vi "LET Output.vi"() -> ()   [LabVIEW 2010]
doc: "Cont(inuous) Acq(uire) & Chart (hw timed) demonstrates the hardware timed, non-buffered technique of data acquisition. The scan clock on the board controls acquisition timing. Acquired scans are read directly from the device's FIFO using AI Single Scan. \n\nThe acquisition is configured with no buffer, and the on-board scan clock started at the selected scan rate. In the first loop iteration, the newest (most recent) scan is read from the FIFO. In each subsequent loop iteration AI Single Scan is called to read the oldest scan from the FIFO. Then if a scan is missed because the acquisition does not keep up, an error message will be displayed, and the acquisition stopped. Each scan is plotted on the chart after it is read. \n\nA common reason to use non-buffered acquisition is that some kind of processing needs to be done for each data point. You will probably want to add more functions to the diagram to customize this VI for your application. The acquisition rate you can achieve depends on how much processing and display the VI must do. This VI calls a subVI named My Single-Scan Processing. Add whatever processing you need to this subVI, or replace it with one of your own. The data processing subVI also demonstrates how to use error clusters in your own subVIs, so they can be included in the error data flow chain.\n\nBefore running this VI, set the values of the controls on the front panel. Select Show Help Window from the Help menu to see a description of each control. If the values you select for all the controls are values you will usually use, select Make Current Values Default from the Operate menu and save the VI. Or, you may save individual control's default values by popping up on the control, selecting Data Operations, then selecting Make Current Value Default, and saving the VI."
uses:
  <instrlib>/agilent_b2900_series/Agilent B2900 Series/Public/Configure/Measurement/Configure Measurement (Current).vi
  <instrlib>/agilent_b2900_series/Agilent B2900 Series/Public/Configure/Measurement/Configure Measurement (Voltage).vi
  <vilib>/Analysis/Matrix/Numeric/Conversions/Matrix To Array - RM.vi
  <vilib>/Utility/file.llb/Write To Spreadsheet File (DBL).vi
  <vilib>/Utility/file.llb/Write To Spreadsheet File (string).vi
  <instrlib>/agilent_b2900_series/Agilent B2900 Series/Agilent B2900 Series.lvlib
  <vilib>/Analysis/Matrix/NI_Matrix.lvlib
panel:
  in  "File Name":string
  in  "WithTimeStamp":bool
  in  "File path":path
  in  "AutoSave":bool
  out "header":string[](array[string])
  out "Real 2D Array":dbl[][](array[numeric])
  out "data matrix":dbl[][](array[numeric])
  out "Igs array 2":dbl[][](array[numeric])
  out "Vgs array 2":dbl[][](array[numeric])
  out "Vds array 2":dbl[][](array[numeric])
  out "Corrected PD current array 2":dbl[][](array[numeric])
  out "Ids array 2":dbl[][](array[numeric])
  out "corrected PD current array":dbl[](array[numeric])
  out "Vds array":dbl[](array[numeric])
  out "Ids array":dbl[](array[numeric])
  out "Vgs array":dbl[](array[numeric])
  out "Igs array":dbl[](array[numeric])
  in  "Tab Control":T1(tab)
  in  "keithley address":string="GPIB0::20::INSTR"
  in  "agilent address":refnum<visa-resource-name>="GPIB0::23::INSTR"
  in  "Initial Vds (V)\n(100 scans/sec)":sgl caption="Initial Vds (V)" format="%.2f"
  in  "Vds step (V)":sgl=1.0 format="%.2f"
  in  "Vds delay time":sgl=10.0 caption="Vds delay time (ms)" format="%.2f"
  in  "Vds delay after first value (ms)":sgl=10.0 format="%.2f"
  in  "Final Vds(V)":sgl=60.0 format="%.2f"
  in  "light emission ON/OFF":bool=TRUE
  in  "Vgs step (V)":sgl=20.0 format="%.2f"
  in  "Final Vgs (V)":sgl=60.0 format="%.2f"
  in  "Initial Vgs (V)":sgl format="%.2f"
  in  "Vgs hold time (ms)":i32=10
  in  "Compliance Voltage (channel 2)":dbl=60.0
  in  "Compliance Current (channel 1)":dbl=0.001
  in  "Compliance Voltage (channel 1)":dbl=60.0
  in  "Compliance Current (channel 2)":dbl=0.0001
  in  "keithley compliance limit":dbl(ring)=0.025 items=["25uA"=2.5e-05, "250uA"=0.00025, "2.5mA"=0.0025, "25mA"=0.025]
  in  "Loop":bool=TRUE
  in  "keithley current resolution":dbl=0.01 format="%^.2e"
  in  "Current Auto Range Mode (0: Normal)":i32(ring) items=["Normal", "Resolution", "Speed"]
  in  "Voltage Auto Range Mode (0: Normal)":i32(ring) items=["Normal", "Resolution", "Speed"]
  out "Current Scan":cluster{dbl[], dbl[]}(graph)
  out "Applied Vds":sgl caption="current VDS (V)" format="%.2f"
  out "Applied Vgs":sgl caption="current VDS (V)" format="%.2f"
  out "Measured Ids":dbl format="%.2e"
  out "Measured Vds":dbl
  out "corrected PD current":dbl format="%^.2e"
  out "dark PD current (A)":dbl format="%^.2e"
  out "PD current":dbl format="%^.2e"
  out "Measured Igs":dbl
  out "Measured Vgs":dbl
  out "channel 2 status":bool
  out "channel 1 status":bool
  out "Current Scan 2":cluster{dbl[], dbl[]}(graph) caption="Current Scan"
  out "half  points":sgl
  out "Vds points":sgl
  out "Vgs points":sgl
  out "?":cluster{dbl[], dbl[]}[](graph)
  out "?":cluster{dbl[], dbl[]}[](graph)
  in  "error in keithley":errorcluster
  out "keithley address out":refnum<k15>
  out "error out keithley":errorcluster
  out "error out agilent":errorcluster
  out "Agilent address out":refnum<visa-resource-name>
  # "FET output v3"
  # "Drain-Source Setting"
  # "Gate Setting"
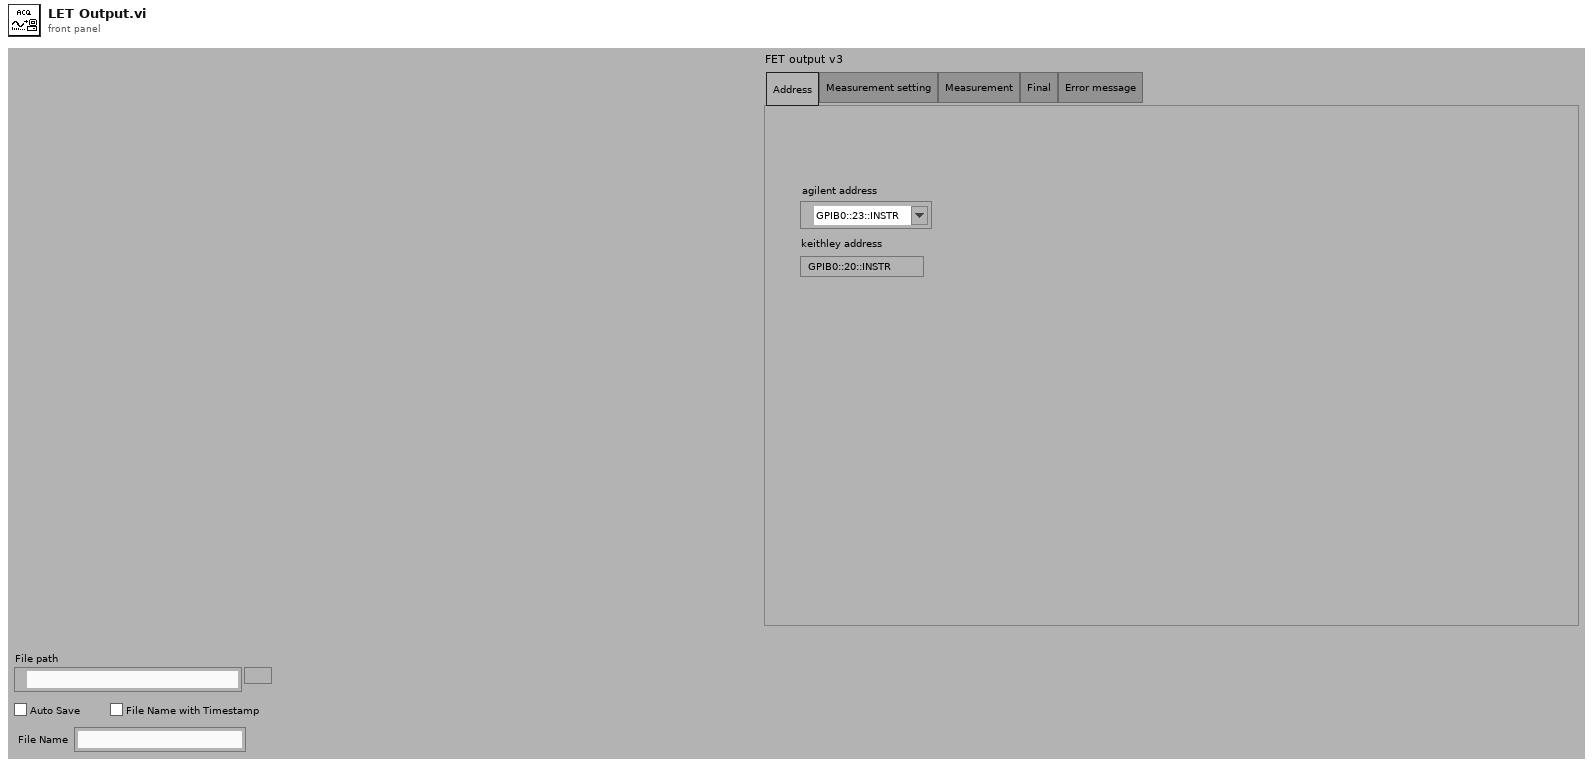
[diagram p1: front panel]
types:
  T1 = enum32{"Address", "Measurement setting", "Measurement", "Final", "Error message"}
  T2 = typedef "NI_Matrix.lvlib/RealMatrix.ctl" = dbl[][]
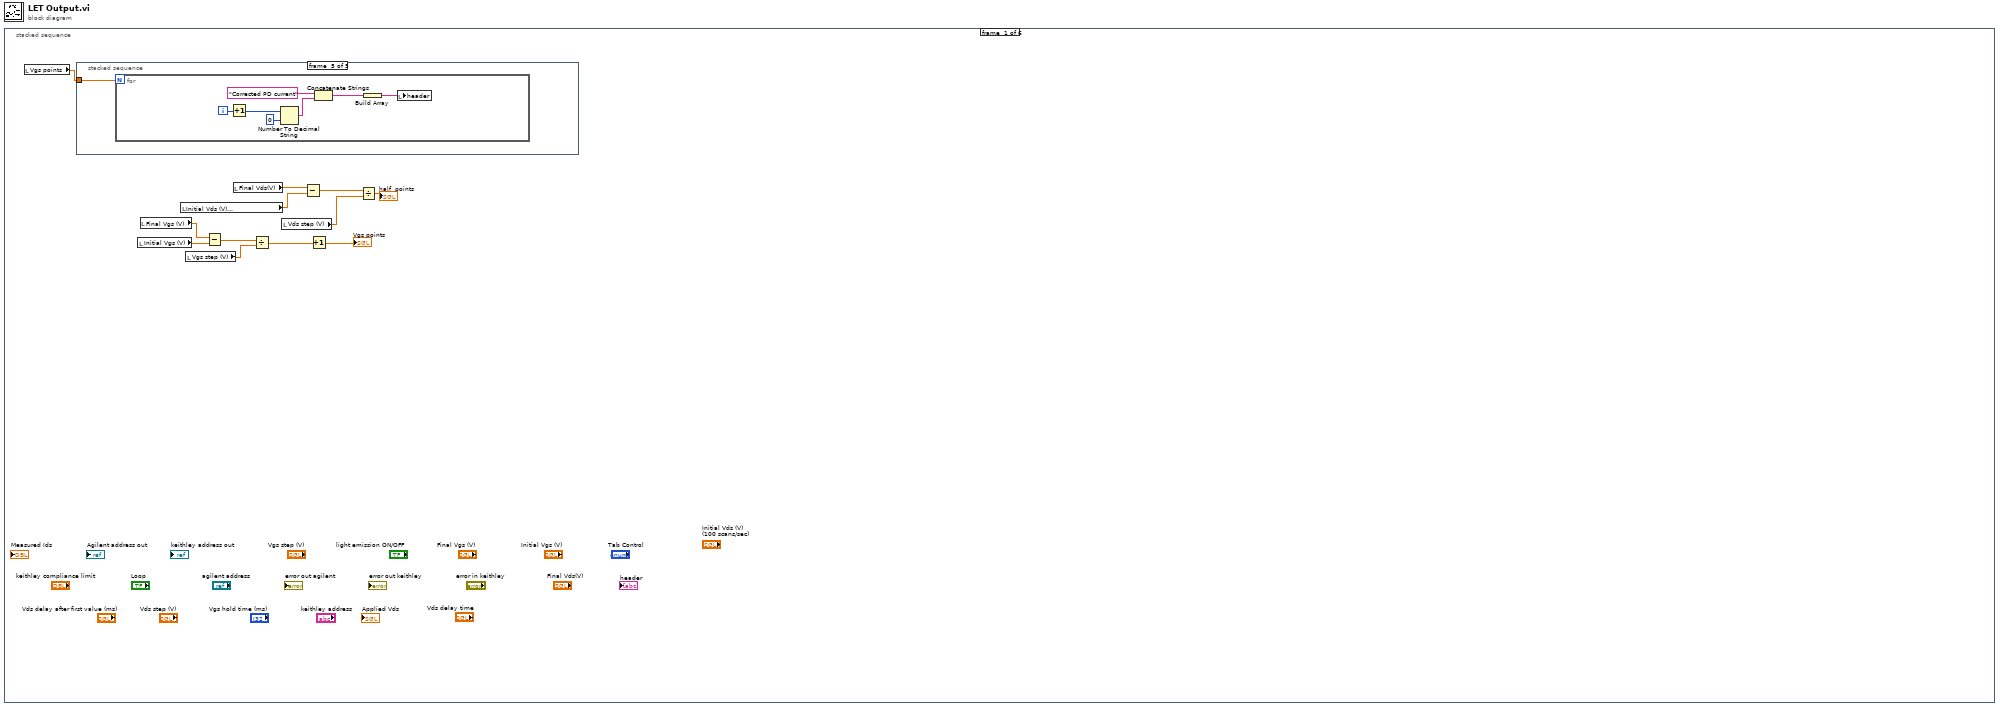
[diagram p0: block diagram]
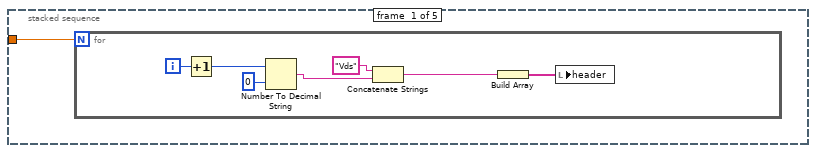
[diagram p2: hidden frame]
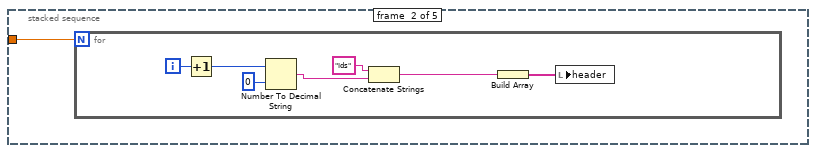
[diagram p3: hidden frame]
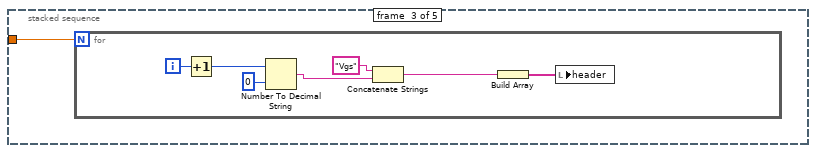
[diagram p4: hidden frame]
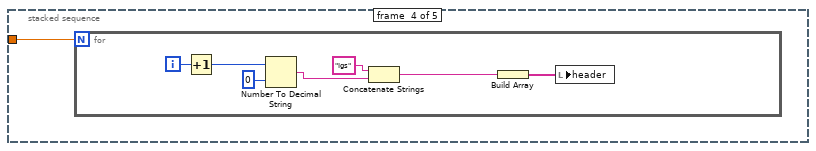
[diagram p5: hidden frame]
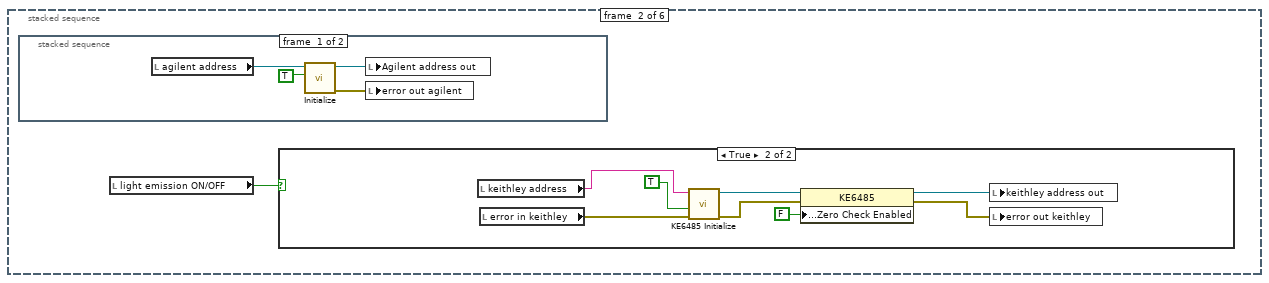
[diagram p6: hidden frame]
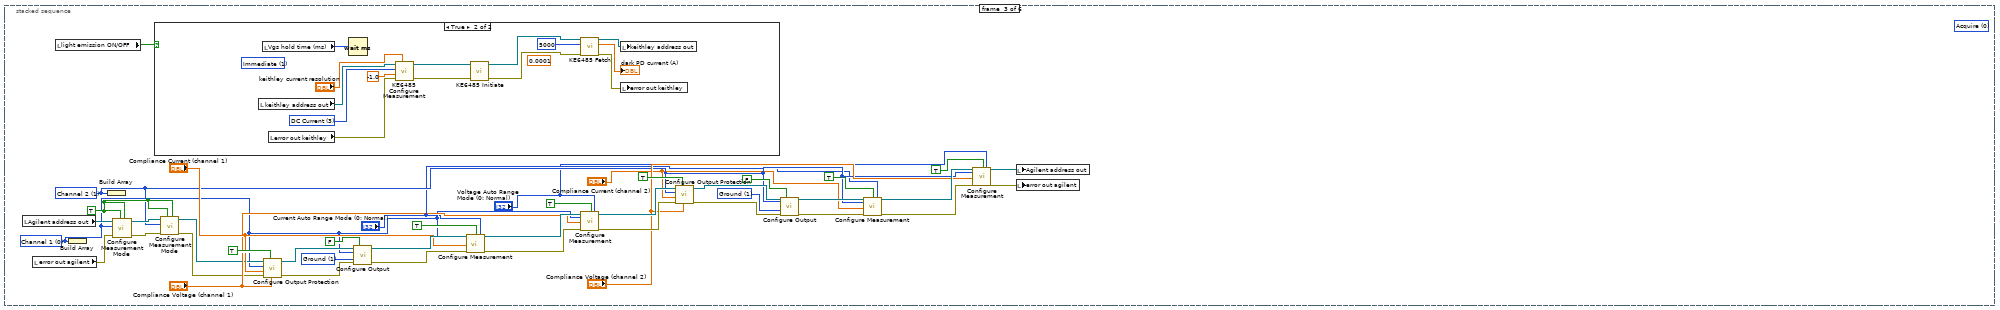
[diagram p9: hidden frame]
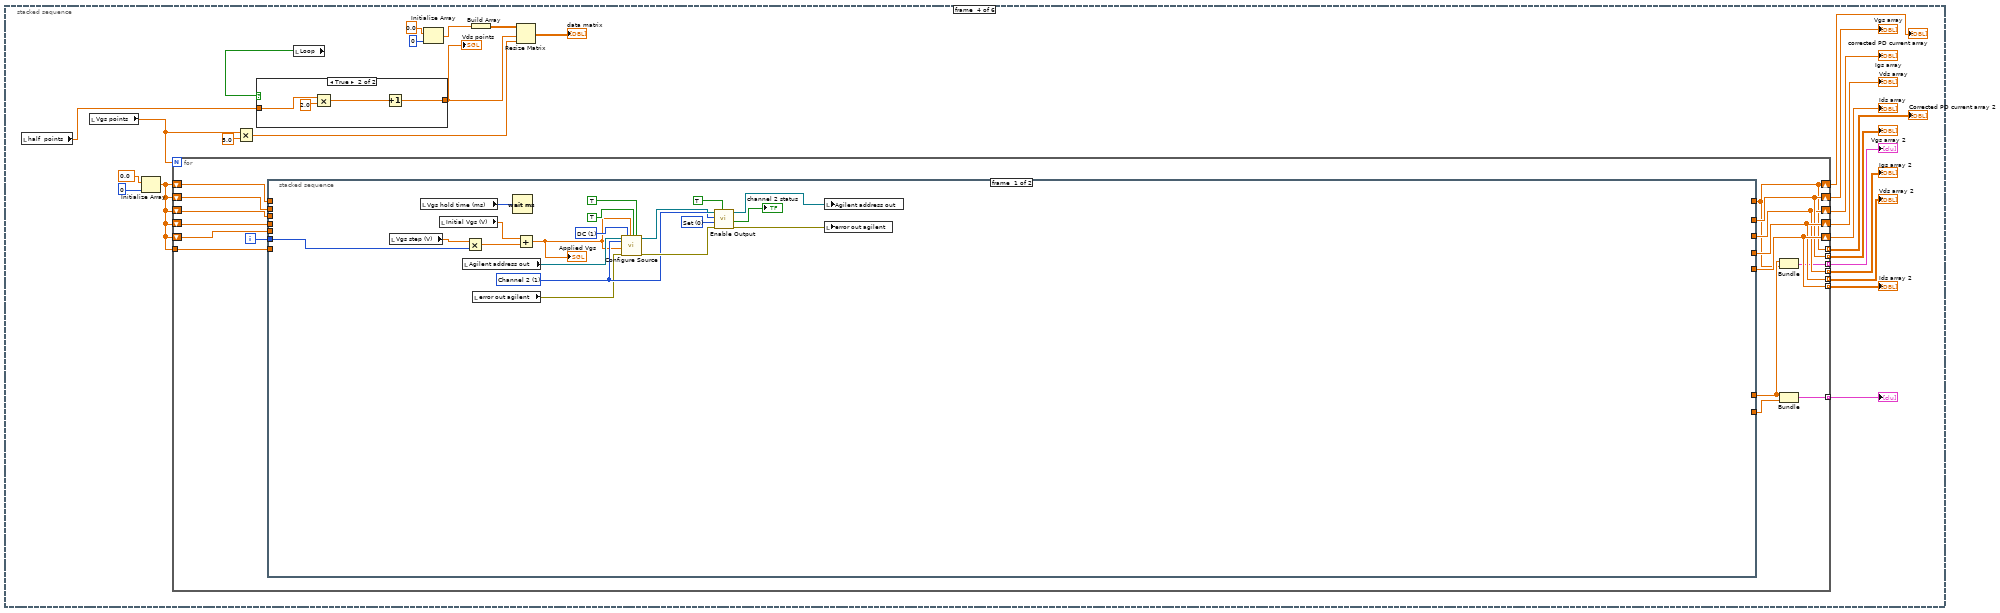
[diagram p11: hidden frame]
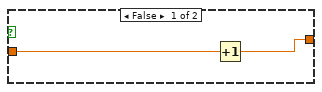
[diagram p12: hidden frame]
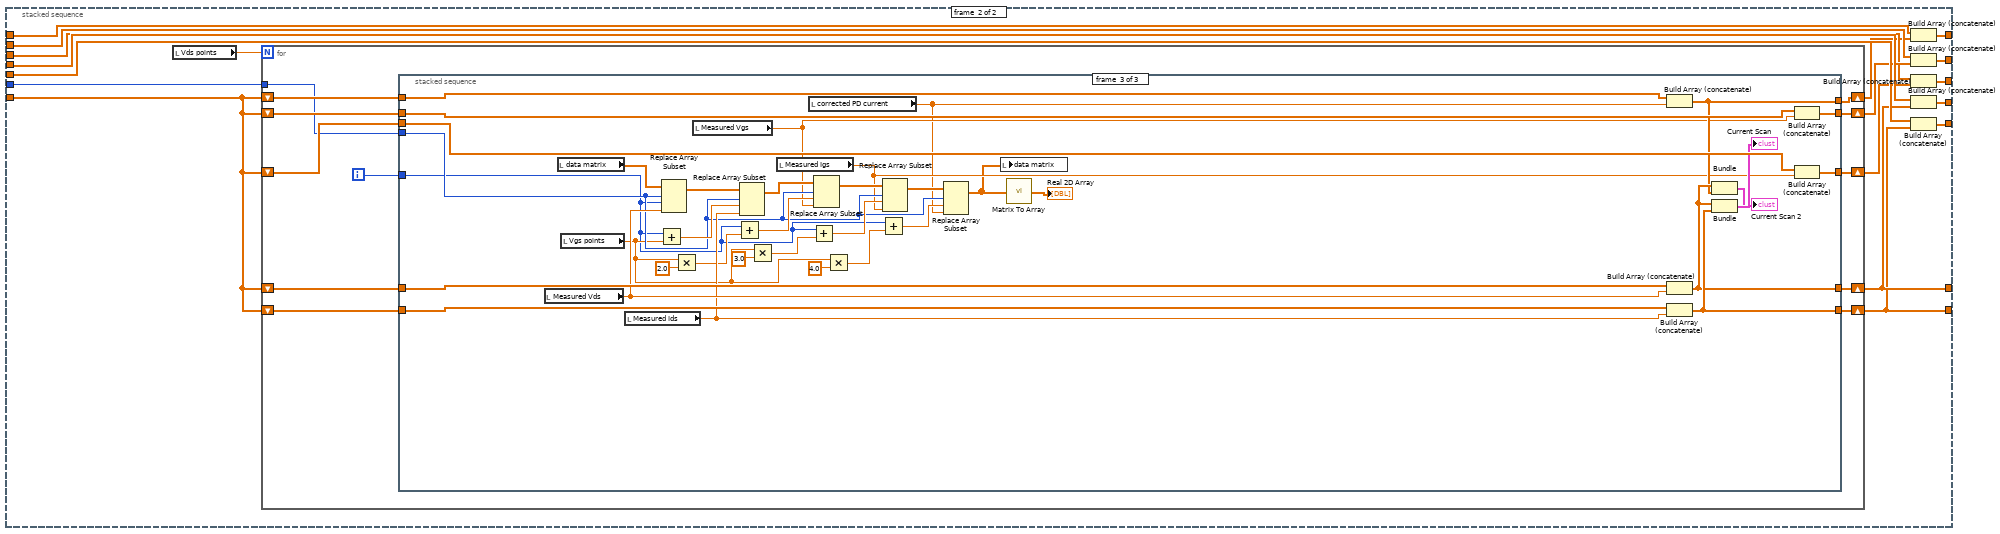
[diagram p13: hidden frame]
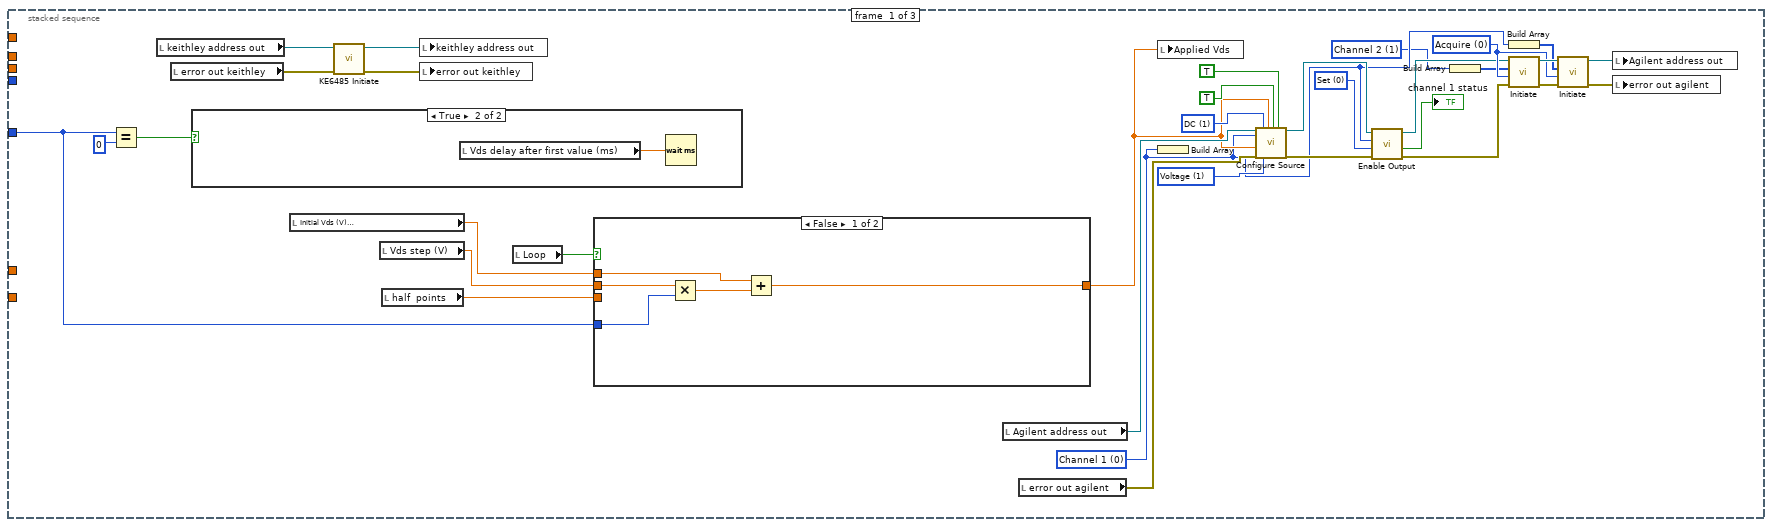
[diagram p14: hidden frame]
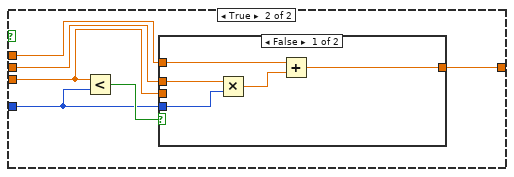
[diagram p15: hidden frame]
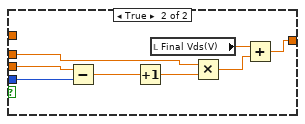
[diagram p16: hidden frame]
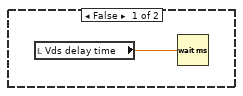
[diagram p17: hidden frame]
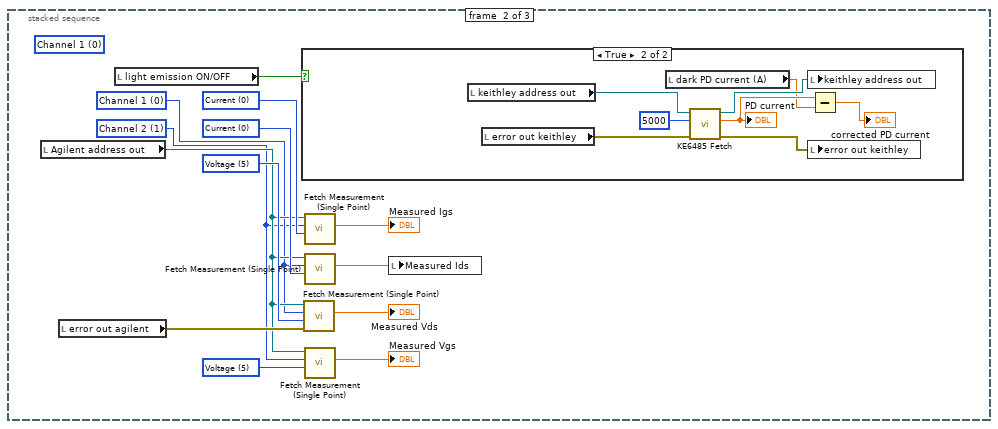
[diagram p18: hidden frame]
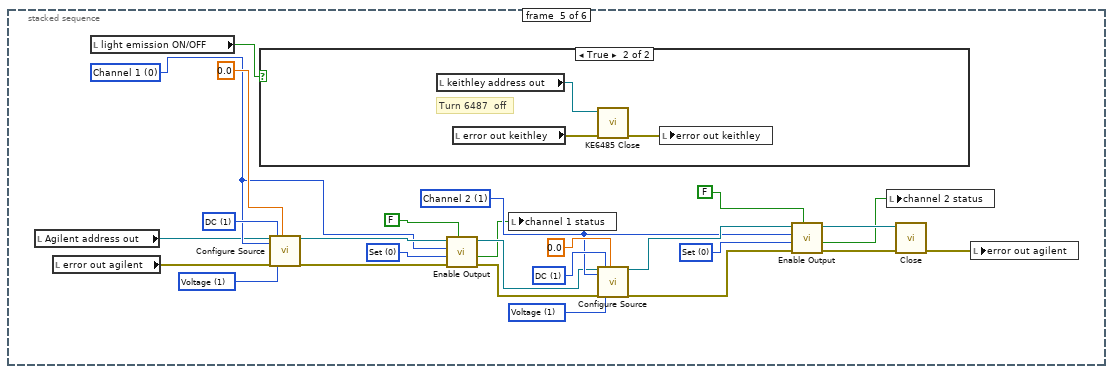
[diagram p20: hidden frame]
diagram:
  n1 = stacked-sequence {
    frame #0 {
      n2 = local read "Vgs points"() -> (w12:sgl)
      n3 = stacked-sequence {
        tunnel: w12 -> [w13 w21 w29 w37 w45]
        frame #0 {
          n4 = for {
            N: w13 -> [_]
            i -> [w20]
            n5 = Increment(x=w20) -> (x+1=w19:i32)
            n6 = Number To Decimal String(number=w19, width (-)=i16 0) -> (decimal integer string=w16:string)
            n7 = Concatenate Strings("Vds" ("delimiter (\\t)"), w16) -> (w17:string)
            n8 = Build Array(w17) -> (w14:string[])
            n9 = local write "header"(w14) -> ()
          }
        }
        frame #1 {
          n10 = for {
            N: w21 -> [_]
            i -> [w28]
            n11 = Increment(x=w28) -> (x+1=w27:i32)
            n12 = Number To Decimal String(number=w27, width (-)=i16 0) -> (decimal integer string=w24:string)
            n13 = Concatenate Strings("Ids" ("delimiter (\\t)"), w24) -> (w25:string)
            n14 = Build Array(w25) -> (w22:string[])
            n15 = local write "header"(w22) -> ()
          }
        }
        frame #2 {
          n16 = for {
            N: w29 -> [_]
            i -> [w36]
            n17 = Increment(x=w36) -> (x+1=w35:i32)
            n18 = Number To Decimal String(number=w35, width (-)=i16 0) -> (decimal integer string=w32:string)
            n19 = Concatenate Strings("Vgs" ("delimiter (\\t)"), w32) -> (w33:string)
            n20 = Build Array(w33) -> (w30:string[])
            n21 = local write "header"(w30) -> ()
          }
        }
        frame #3 {
          n22 = for {
            N: w37 -> [_]
            i -> [w44]
            n23 = Increment(x=w44) -> (x+1=w43:i32)
            n24 = Number To Decimal String(number=w43, width (-)=i16 0) -> (decimal integer string=w40:string)
            n25 = Concatenate Strings("Igs" ("delimiter (\\t)"), w40) -> (w41:string)
            n26 = Build Array(w41) -> (w38:string[])
            n27 = local write "header"(w38) -> ()
          }
        }
        frame #4 {
          n28 = for {
            N: w45 -> [_]
            i -> [w52]
            n29 = Increment(x=w52) -> (x+1=w51:i32)
            n30 = Number To Decimal String(number=w51, width (-)=i16 0) -> (decimal integer string=w48:string)
            n31 = Concatenate Strings("Corrected PD current" ("delimiter (\\t)"), w48) -> (w49:string)
            n32 = Build Array(w49) -> (w46:string[])
            n33 = local write "header"(w46) -> ()
          }
        }
      }
      n34 = local read "Initial Vgs (V)"() -> (w6:sgl)
      n35 = local read "Final Vgs (V)"() -> (w5:sgl)
      n36 = local read "Initial Vds (V)\n(100 scans/sec)"() -> (w9:sgl)
      n37 = local read "Vgs step (V)"() -> (w7:sgl)
      n38 = Subtract(x=w5, y=w6) -> (x-y=w3:sgl)
      n39 = local read "Final Vds(V)"() -> (w8:sgl)
      n40 = Divide(x=w3, y=w7) -> (x/y=w4:sgl)
      n41 = local read "Vds step (V)"() -> (w10:sgl)
      n42 = Subtract(x=w8, y=w9) -> (x-y=w11:sgl)
      n43 = Increment(x=w4) -> (x+1=→"Vgs points":sgl)
      n44 = Divide(x=w11, y=w10) -> (x/y=→"half  points":sgl)
    }
    frame #1 {
      n45 = stacked-sequence {
        frame #0 {
          n46 = local read "agilent address"() -> (w54:refnum<visa-resource-name>)
          n47 = call <instrlib>:"Initialize.vi"("ID Query (True)"=TRUE, "VISA resource name"=w54) -> ("error out"=w55:errorcluster, "VISA resource name out"=w56:refnum<visa-resource-name>)  [unwired: 8 in]
          n48 = local write "Agilent address out"(w56) -> ()
          n49 = local write "error out agilent"(w55) -> ()
        }
        frame #1 {
        }
      }
      n50 = local read "light emission ON/OFF"() -> (w53:bool)
      n51 = case shown="True" w53 {
        frame False {
        }
        frame True {
          n52 = local read "keithley address"() -> (w64:string)
          n53 = local read "error in keithley"() -> (w65:errorcluster)
          n54 = call <instrlib>:"KE6485 Initialize.vi"("error in (no error)"=w65, "reset device"=TRUE, "resource name"=w64) -> ("error out"=w62:errorcluster, "instrument handle out"=w61:refnum<k15>)  [unwired: 1 in, 6 out]
          n55 = property class="KE6485"(reference=w61, error in=w62, "System Settings:Zero Check Enabled"=FALSE) -> (reference out=w60:refnum<k15>, error out=w59:errorcluster)
          n56 = local write "keithley address out"(w60) -> ()
          n57 = local write "error out keithley"(w59) -> ()
        }
      }
    }
    frame #2 {
      (unwired) 0 items=["Acquire", "Transient", "Both"] ("Device Action (2: Both)")
      w78 = TRUE ("Enable Voltage Measurement (T: Enable)")
      w90 = 1 items=["Float", "Ground"] ("Low Terminal State (1: Ground)")
      w70 = 1 items=["Channel 1", "Channel 2"] ("Channel (0: Channel 1)")
      w100 = 1 items=["Float", "Ground"] ("Low Terminal State (1: Ground)")
      w71 = 0 items=["Channel 1", "Channel 2"] ("Channel (0: Channel 1)")
      n58 = local read "Agilent address out"() -> (w73:refnum<visa-resource-name>)
      n59 = local read "error out agilent"() -> (w75:errorcluster)
      n60 = local read "light emission ON/OFF"() -> (w107:bool)
      n61 = Build Array(w71) -> ()  [unwired: 1 out]
      n62 = Build Array(w70) -> ()  [unwired: 1 out]
      n63 = call <instrlib>:"Configure Measurement Mode.vi"("Enable Current Measurement (T: Enable)"=w78, "Enable Voltage Measurement (T: Enable)"=w78, "error in (no error)"=w75, "Channel (0: Channel 1)"=w71, "VISA resource name"=w73) -> ("error out"=w76:errorcluster, "VISA resource name out"=w77:refnum<visa-resource-name>)  [unwired: 5 in]
      n64 = case shown="True" w107 {
        frame False {
        }
        frame True {
          (unwired) 0.0001 ("resolution (absolute)")
          (unwired) 1 items=["Immediate"=1, "Interval"=10, "Trigger Link 1"=1001, "Trigger Link 2"=1002, "Trigger Link 3"=1003, "Trigger Link 4"=1004, "Trigger Link 5"=1005, "Trigger Link 6"=1006] ("sample trigger")
          w119 = 3 items=["DC Volts"=1, "DC Current"=3, "2 Wire Resistance"=5, "Charge"=1004] ("measurement function")
          n65 = local read "keithley address out"() -> (w114:refnum<k15>)
          n66 = local read "Vgs hold time (ms)"() -> (w121:i32)
          n67 = local read "error out keithley"() -> (w113:errorcluster)
          n68 = Wait (ms)(milliseconds to wait=w121) -> ()  [unwired: 1 out]
          n69 = call <instrlib>:"KE6485 Configure Measurement.vi"("resolution (absolute)"="keithley current resolution", "error in (no error)"=w113, "range"=-1.0, "measurement function"=w119, "instrument handle"=w114) -> ("error out"=w110:errorcluster, "instrument handle out"=w112:refnum<k15>)  [unwired: 5 in]
          n70 = call <instrlib>:"KE6485 Initiate.vi"("error in (no error)"=w110, "instrument handle"=w112) -> ("error out"=w109:errorcluster, "instrument handle out"=w111:refnum<k15>)  [unwired: 8 in]
          n71 = call <instrlib>:"KE6485 Fetch.vi"("error in (no error)"=w109, "maximum time (ms)"=5000, "instrument handle"=w111) -> ("error out"=w116:errorcluster, "reading"=→"dark PD current (A)":dbl, "instrument handle out"=w115:refnum<k15>)  [unwired: 6 in]
          n72 = local write "keithley address out"(w115) -> ()
          n73 = local write "error out keithley"(w116) -> ()
        }
      }
      n74 = call <instrlib>:"Configure Measurement Mode.vi"("Enable Current Measurement (T: Enable)"=w78, "Enable Voltage Measurement (T: Enable)"=w78, "error in (no error)"=w76, "Channel (0: Channel 1)"=w70, "VISA resource name"=w77) -> ("error out"=w74:errorcluster, "VISA resource name out"=w72:refnum<visa-resource-name>)  [unwired: 5 in]
      n75 = call <instrlib>:"Configure Output Protection.vi"("Compliance Voltage (2 V)"="Compliance Voltage (channel 1)", "Enable Output Protection (T: Enable)"=TRUE, "error in (no error)"=w74, "Compliance Current (0.0001 A)"="Compliance Current (channel 1)", "Channel (0: Channel 1)"=w71, "VISA resource name"=w72) -> ("error out"=w102:errorcluster, "VISA resource name out"=w101:refnum<visa-resource-name>)  [unwired: 4 in]
      n76 = call <instrlib>:"Configure Output.vi"("VISA resource name"=w101, "Auto Output-Off (F: Disable)"=FALSE, "Channel (0: Channel 1)"=w71, "Low Terminal State (1: Ground)"=w100, "error in (no error)"=w102) -> ("VISA resource name out"=w98:refnum<visa-resource-name>, "error out"=w99:errorcluster)  [unwired: 9 in]
      n77 = call-poly <instrlib>:"Configure Measurement.vi"("VISA resource name"=w98, "Channel (0: Channel 1)"=w71, "Current Range (0.0001 A)"="Compliance Current (channel 1)", "error in (no error)"=w99, "Current Auto Range (T: Enable)"=TRUE, "Current Auto Range Mode (0: Normal)"="Current Auto Range Mode (0: Normal)") -> ("VISA resource name out"=w106:refnum<visa-resource-name>, "error out"=w105:errorcluster)  [unwired: 12 in]
      n78 = call-poly <instrlib>:"Configure Measurement.vi"("VISA resource name"=w106, "Channel (0: Channel 1)"=w71, "Voltage Range (2 V)"="Compliance Voltage (channel 1)", "error in (no error)"=w105, "Voltage Auto Range (T: Enable)"=TRUE, "Voltage Auto Range Mode (0: Normal)"="Voltage Auto Range Mode (0: Normal)") -> ("VISA resource name out"=w86:refnum<visa-resource-name>, "error out"=w85:errorcluster)  [unwired: 12 in]
      n79 = call <instrlib>:"Configure Output Protection.vi"("Compliance Voltage (2 V)"="Compliance Voltage (channel 2)", "Enable Output Protection (T: Enable)"=TRUE, "error in (no error)"=w85, "Compliance Current (0.0001 A)"="Compliance Current (channel 2)", "Channel (0: Channel 1)"=w70, "VISA resource name"=w86) -> ("error out"=w92:errorcluster, "VISA resource name out"=w91:refnum<visa-resource-name>)  [unwired: 4 in]
      n80 = call <instrlib>:"Configure Output.vi"("VISA resource name"=w91, "Auto Output-Off (F: Disable)"=FALSE, "Channel (0: Channel 1)"=w70, "Low Terminal State (1: Ground)"=w90, "error in (no error)"=w92) -> ("VISA resource name out"=w88:refnum<visa-resource-name>, "error out"=w89:errorcluster)  [unwired: 9 in]
      n81 = call-poly <instrlib>:"Configure Measurement.vi"("VISA resource name"=w88, "Channel (0: Channel 1)"=w70, "Current Range (0.0001 A)"="Compliance Current (channel 2)", "error in (no error)"=w89, "Current Auto Range (T: Enable)"=TRUE, "Current Auto Range Mode (0: Normal)"="Current Auto Range Mode (0: Normal)") -> ("VISA resource name out"=w96:refnum<visa-resource-name>, "error out"=w95:errorcluster)  [unwired: 12 in]
      n82 = call-poly <instrlib>:"Configure Measurement.vi"("VISA resource name"=w96, "Channel (0: Channel 1)"=w70, "Voltage Range (2 V)"="Compliance Voltage (channel 2)", "error in (no error)"=w95, "Voltage Auto Range (T: Enable)"=TRUE, "Voltage Auto Range Mode (0: Normal)"="Voltage Auto Range Mode (0: Normal)") -> ("VISA resource name out"=w69:refnum<visa-resource-name>, "error out"=w68:errorcluster)  [unwired: 12 in]
      n83 = local write "Agilent address out"(w69) -> ()
      n84 = local write "error out agilent"(w68) -> ()
    }
    frame #3 {
      n85 = local read "half  points"() -> (w122:sgl)
      n86 = local read "Vgs points"() -> (w123:sgl)
      n87 = Initialize Array(0.0, 0) -> (w138:dbl[])
      n88 = for {
        N: w123 -> [_]
        shift-right: [w160] -> w144
        shift-left: w138 -> [w168]
        shift-right: [w161] -> w145
        shift-left: w138 -> [w167]
        shift-right: [w158] -> w143
        shift-left: w138 -> [w166]
        tunnel: [w165] -> w142 mode=indexing
        shift-right: [w157] -> w140
        shift-left: w138 -> [w164]
        shift-right: [w155] -> w139
        shift-left: w138 -> [w163]
        tunnel: w138 -> [w162]
        tunnel: [w161] -> w137 mode=indexing
        tunnel: [w155] -> w136 mode=indexing
        tunnel: [w160] -> w135 mode=indexing
        tunnel: [w158] -> w134 mode=indexing
        tunnel: [w157] -> w133 mode=indexing
        tunnel: [w154] -> w132 mode=indexing
        i -> [w169]
        n89 = stacked-sequence {
          tunnel: w169 -> [w184 w189]
          tunnel: w168 -> [_ w206]
          tunnel: w167 -> [_ w205]
          tunnel: [_ w200] -> w160
          tunnel: [_ w204] -> w161
          tunnel: w166 -> [_ w202]
          tunnel: [_ w201] -> w158
          tunnel: [_ w199] -> w156
          tunnel: [_ w198] -> w159
          tunnel: w164 -> [_ w197]
          tunnel: [_ w196] -> w157
          tunnel: [_ w194] -> w155
          tunnel: w163 -> [_ w192]
          tunnel: w162 -> [_ w190]
          frame #0 {
            w177 = 0 items=["Set", "Get"] ("Operation (0: Set)")
            w178 = 1 items=["Channel 1", "Channel 2"] ("Channel (0: Channel 1)")
            w181 = 1 items=["Pulse", "DC"] ("Source Shape (1: DC)")
            n90 = local read "Vgs step (V)"() -> (w188:sgl)
            n91 = local read "Vgs hold time (ms)"() -> (w186:i32)
            n92 = local read "Initial Vgs (V)"() -> (w187:sgl)
            n93 = local read "Agilent address out"() -> (w174:refnum<visa-resource-name>)
            n94 = Multiply(x=w188, y=w184) -> (x*y=w185:sgl)
            n95 = local read "error out agilent"() -> (w173:errorcluster)
            n96 = Wait (ms)(milliseconds to wait=w186) -> ()  [unwired: 1 out]
            n97 = Add(x=w187, y=w185) -> (x+y=w170:sgl)
            "Applied Vgs" <- w170
            n98 = call <instrlib>:"Configure Source.vi"("VISA resource name"=w174, "Channel (0: Channel 1)"=w178, "Source Range (2)"=w170, "error in (no error)"=w173, "Source Shape (1: DC)"=w181, "Output Level (0)"=w170, "Source Auto Range (T: Enable)"=TRUE, "Enable Continuous Output (T: Enable)"=TRUE) -> ("VISA resource name out"=w183:refnum<visa-resource-name>, "error out"=w182:errorcluster)  [unwired: 10 in]
            n99 = call <instrlib>:"Enable Output.vi"("Enable Output (T: Enable)"=TRUE, "error in (no error)"=w182, "Operation (0: Set)"=w177, "Channel (0: Channel 1)"=w178, "VISA resource name"=w183) -> ("error out"=w172:errorcluster, "Output Enabled?"=→"channel 2 status":bool, "VISA resource name out"=w171:refnum<visa-resource-name>)  [unwired: 4 in]
            n100 = local write "Agilent address out"(w171) -> ()
            n101 = local write "error out agilent"(w172) -> ()
          }
          frame #1 {
            n102 = local read "Vds points"() -> (w191:sgl)
            n103 = for {
              N: w191 -> [_]
              shift-right: [w209] -> w198
              shift-left: w190 -> [w208]
              shift-right: [w211] -> w199
              shift-left: w190 -> [w210]
              shift-right: [w215] -> w203
              shift-left: w190 -> [w214]
              shift-right: [w213] -> w195
              shift-left: w190 -> [w212]
              shift-right: [w216] -> w193
              shift-left: w190 -> [w217]
              tunnel: w189 -> [w207]
              i -> [w218]
              n104 = stacked-sequence {
                tunnel: w218 -> [w238 _ w301]
                tunnel: w217 -> [_ _ w335]
                tunnel: [_ _ w324] -> w216
                tunnel: [_ _ w334] -> w215
                tunnel: w214 -> [_ _ w333]
                tunnel: [_ _ w332] -> w213
                tunnel: w212 -> [_ _ w331]
                tunnel: [_ _ w325] -> w211
                tunnel: w210 -> [_ _ w329]
                tunnel: [_ _ w327] -> w209
                tunnel: w208 -> [_ _ w328]
                tunnel: w207 -> [_ _ w309]
                frame #0 {
                  w231 = 0 items=["Acquire", "Transient", "Both"] ("Device Action (2: Both)")
                  w223 = 1 items=["Channel 1", "Channel 2"] ("Channel (0: Channel 1)")
                  w240 = 1 items=["Current", "Voltage"] ("Source Mode (1: Voltage)")
                  w243 = 1 items=["Pulse", "DC"] ("Source Shape (1: DC)")
                  w224 = 0 items=["Channel 1", "Channel 2"] ("Channel (0: Channel 1)")
                  w247 = 0 items=["Set", "Get"] ("Operation (0: Set)")
                  n105 = Equal?(x=w238, y=0) -> (x = y?=w250:bool)
                  n106 = local read "keithley address out"() -> (w220:refnum<k15>)
                  n107 = local read "error out keithley"() -> (w219:errorcluster)
                  n108 = case shown="True" w250 {
                    frame False {
                      n109 = local read "Vds delay time"() -> (w276:sgl)
                      n110 = Wait (ms)(milliseconds to wait=w276) -> ()  [unwired: 1 out]
                    }
                    frame True {
                      n111 = local read "Vds delay after first value (ms)"() -> (w277:sgl)
                      n112 = Wait (ms)(milliseconds to wait=w277) -> ()  [unwired: 1 out]
                    }
                  }
                  n113 = local read "Initial Vds (V)\n(100 scans/sec)"() -> (w239:sgl)
                  n114 = call <instrlib>:"KE6485 Initiate.vi"("error in (no error)"=w219, "instrument handle"=w220) -> ("error out"=w222:errorcluster, "instrument handle out"=w221:refnum<k15>)  [unwired: 8 in]
                  n115 = local read "Vds step (V)"() -> (w237:sgl)
                  n116 = local read "half  points"() -> (w235:sgl)
                  n117 = local write "keithley address out"(w221) -> ()
                  n118 = local write "error out keithley"(w222) -> ()
                  n119 = local read "Loop"() -> (w236:bool)
                  n120 = case shown="False" w236 {
                    tunnel: [w255 w261] -> w234
                    tunnel: w238 -> [w254 w258]
                    tunnel: w239 -> [w253 w260]
                    tunnel: w237 -> [w252 w259]
                    tunnel: w235 -> [_ w257]
                    frame False {
                      n121 = Multiply(x=w252, y=w254) -> (x*y=w256:sgl)
                      n122 = Add(x=w253, y=w256) -> (x+y=w255:sgl)
                    }
                    frame True {
                      n123 = Less?(x=w257, y=w258) -> (x < y?=w262:bool)
                      n124 = case shown="False" w262 {
                        tunnel: [w266 w275] -> w261
                        tunnel: w260 -> [w265 _]
                        tunnel: w258 -> [w264 w272]
                        tunnel: w259 -> [w263 w273]
                        tunnel: w257 -> [_ w271]
                        frame False {
                          n125 = Multiply(x=w263, y=w264) -> (x*y=w267:sgl)
                          n126 = Add(x=w265, y=w267) -> (x+y=w266:sgl)
                        }
                        frame True {
                          n127 = Subtract(x=w271, y=w272) -> (x-y=w269:sgl)
                          n128 = Increment(x=w269) -> (x+1=w268:sgl)
                          n129 = local read "Final Vds(V)"() -> (w270:sgl)
                          n130 = Multiply(x=w273, y=w268) -> (x*y=w274:sgl)
                          n131 = Add(x=w270, y=w274) -> (x+y=w275:sgl)
                        }
                      }
                    }
                  }
                  n132 = local read "Agilent address out"() -> (w245:refnum<visa-resource-name>)
                  n133 = local read "error out agilent"() -> (w244:errorcluster)
                  n134 = local write "Applied Vds"(w234) -> ()
                  n135 = Build Array(w224) -> ()  [unwired: 1 out]
                  n136 = call <instrlib>:"Configure Source.vi"("VISA resource name"=w245, "Channel (0: Channel 1)"=w224, "Source Range (2)"=w234, "error in (no error)"=w244, "Source Shape (1: DC)"=w243, "Source Mode (1: Voltage)"=w240, "Output Level (0)"=w234, "Source Auto Range (T: Enable)"=TRUE, "Enable Continuous Output (T: Enable)"=TRUE) -> ("VISA resource name out"=w249:refnum<visa-resource-name>, "error out"=w248:errorcluster)  [unwired: 9 in]
                  n137 = call <instrlib>:"Enable Output.vi"("error in (no error)"=w248, "Operation (0: Set)"=w247, "Channel (0: Channel 1)"=w224, "VISA resource name"=w249) -> ("error out"=w227:errorcluster, "Output Enabled?"=→"channel 1 status":bool, "VISA resource name out"=w228:refnum<visa-resource-name>)  [unwired: 5 in]
                  n138 = Build Array(w223) -> (w230:i32[])
                  n139 = Build Array(w224) -> (w229:i32[])
                  n140 = call <instrlib>:"Initiate.vi"("error in (no error)"=w227, "Device Action (2: Both)"=w231, "Channel List ({Channel1})"=w230, "VISA resource name"=w228) -> ("error out"=w233:errorcluster, "VISA resource name out"=w232:refnum<visa-resource-name>)  [unwired: 6 in]
                  n141 = call <instrlib>:"Initiate.vi"("error in (no error)"=w233, "Device Action (2: Both)"=w231, "Channel List ({Channel1})"=w229, "VISA resource name"=w232) -> ("error out"=w226:errorcluster, "VISA resource name out"=w225:refnum<visa-resource-name>)  [unwired: 6 in]
                  n142 = local write "Agilent address out"(w225) -> ()
                  n143 = local write "error out agilent"(w226) -> ()
                }
                frame #1 {
                  w279 = 1 items=["Channel 1", "Channel 2"] ("Channel (0: Channel 1)")
                  w280 = 0 items=["Channel 1", "Channel 2"] ("Channel (0: Channel 1)")
                  w285 = 0 items=["Current", "Resistance", "Source Output Setting", "Status", "Time", "Voltage"] ("Data Mode (5: Voltage)")
                  w286 = 5 items=["Current", "Resistance", "Source Output Setting", "Status", "Time", "Voltage"] ("Data Mode (5: Voltage)")
                  w288 = 0 items=["Current", "Resistance", "Source Output Setting", "Status", "Time", "Voltage"] ("Data Mode (5: Voltage)")
                  (unwired) 0 items=["Channel 1", "Channel 2"] ("Channel (0: Channel 1)")
                  w290 = 5 items=["Current", "Resistance", "Source Output Setting", "Status", "Time", "Voltage"] ("Data Mode (5: Voltage)")
                  n144 = local read "Agilent address out"() -> (w281:refnum<visa-resource-name>)
                  n145 = local read "error out agilent"() -> (w282:errorcluster)
                  n146 = local read "light emission ON/OFF"() -> (w278:bool)
                  n147 = case shown="True" w278 {
                    frame False {
                    }
                    frame True {
                      n148 = local read "keithley address out"() -> (w292:refnum<k15>)
                      n149 = local read "error out keithley"() -> (w291:errorcluster)
                      n150 = local read "dark PD current (A)"() -> (w293:dbl)
                      n151 = call <instrlib>:"KE6485 Fetch.vi"("error in (no error)"=w291, "maximum time (ms)"=5000, "instrument handle"=w292) -> ("error out"=w297:errorcluster, "reading"=w294:dbl, "instrument handle out"=w296:refnum<k15>)  [unwired: 6 in]
                      "PD current" <- w294
                      n152 = local write "keithley address out"(w296) -> ()
                      n153 = local write "error out keithley"(w297) -> ()
                      n154 = Subtract(x=w294, y=w293) -> (x-y=→"corrected PD current":dbl)
                    }
                  }
                  n155 = call <instrlib>:"Fetch Measurement (Single Point).vi"("error in (no error)"=w282, "Data Mode (5: Voltage)"=w290, "Channel (0: Channel 1)"=w280, "VISA resource name"=w281) -> ("Measurement"=→"Measured Vds":dbl)  [unwired: 5 in, 2 out]
                  n156 = call <instrlib>:"Fetch Measurement (Single Point).vi"("Data Mode (5: Voltage)"=w285, "Channel (0: Channel 1)"=w279, "VISA resource name"=w281) -> ("Measurement"=→"Measured Igs":dbl)  [unwired: 6 in, 2 out]
                  n157 = call <instrlib>:"Fetch Measurement (Single Point).vi"("Data Mode (5: Voltage)"=w288, "Channel (0: Channel 1)"=w280, "VISA resource name"=w281) -> ("Measurement"=w287:dbl)  [unwired: 6 in, 2 out]
                  n158 = call <instrlib>:"Fetch Measurement (Single Point).vi"("Data Mode (5: Voltage)"=w286, "Channel (0: Channel 1)"=w279, "VISA resource name"=w281) -> ("Measurement"=→"Measured Vgs":dbl)  [unwired: 6 in, 2 out]
                  n159 = local write "Measured Ids"(w287) -> ()
                }
                frame #2 {
                  n160 = local read "Measured Vds"() -> (w322:dbl)
                  n161 = local read "data matrix"() -> (w323:dbl[][])
                  n162 = local read "Vgs points"() -> (w305:sgl)
                  n163 = local read "Measured Ids"() -> (w319:dbl)
                  n164 = Add(x=w301, y=w305) -> (x+y=w320:sgl)
                  n165 = Replace Array Subset(array=w323, new element=w322, index (row)=w309, index (col)=w301) -> (w321:T2)
                  n166 = Multiply(x=w305, y=sgl 2.0) -> (x*y=w316:sgl)
                  n167 = local read "Measured Vgs"() -> (w304:dbl)
                  n168 = Add(x=w301, y=w316) -> (x+y=w317:sgl)
                  n169 = Replace Array Subset(array=w321, new element=w319, index (row)=w309, index (col)=w320) -> (w318:T2)
                  n170 = Multiply(x=w305, y=sgl 3.0) -> (x*y=w313:sgl)
                  n171 = local read "Measured Igs"() -> (w303:dbl)
                  n172 = local read "corrected PD current"() -> (w302:dbl)
                  n173 = Add(x=w301, y=w313) -> (x+y=w311:sgl)
                  n174 = Replace Array Subset(array=w318, new element=w304, index (row)=w309, index (col)=w317) -> (w314:T2)
                  n175 = Multiply(x=w305, y=sgl 4.0) -> (x*y=w308:sgl)
                  n176 = Add(x=w301, y=w308) -> (x+y=w306:sgl)
                  n177 = Replace Array Subset(array=w314, new element=w303, index (row)=w309, index (col)=w311) -> (w310:T2)
                  n178 = Replace Array Subset(array=w310, new element=w302, index (row)=w309, index (col)=w306) -> (w300:T2)
                  n179 = local write "data matrix"(w300) -> ()
                  n180 = call-poly <vilib>:"Matrix To Array.vi"("Real Matrix"=w300) -> ("Real 2D Array"=→"Real 2D Array":dbl[][])
                  n181 = Build Array (concatenate)(w335, w302) -> (w324:dbl[])
                  n182 = Build Array (concatenate)(w329, w322) -> (w325:dbl[])
                  n183 = Build Array (concatenate)(w328, w319) -> (w327:dbl[])
                  n184 = Bundle(w325, w324) -> (→"Current Scan 2":cluster{dbl[], dbl[]})  [unwired: 1 out]
                  n185 = Bundle(w325, w327) -> (→"Current Scan":cluster{dbl[], dbl[]})  [unwired: 1 out]
                  n186 = Build Array (concatenate)(w333, w304) -> (w334:dbl[])
                  n187 = Build Array (concatenate)(w331, w303) -> (w332:dbl[])
                }
              }
            }
            n188 = Build Array (concatenate)(w192, w193) -> (w194:dbl[])
            n189 = Build Array (concatenate)(w202, w203) -> (w201:dbl[])
            n190 = Build Array (concatenate)(w197, w195) -> (w196:dbl[])
            n191 = Build Array (concatenate)(w206, w199) -> (w200:dbl[])
            n192 = Build Array (concatenate)(w205, w198) -> (w204:dbl[])
          }
        }
        n193 = Bundle(w156, w155) -> (w154:cluster{dbl[], dbl[]})  [unwired: 1 out]
        n194 = Bundle(w156, w159) -> (w165:cluster{dbl[], dbl[]})  [unwired: 1 out]
      }
      "?" <- w142
      "Igs array" <- w140
      "Vgs array" <- w143
      "Ids array" <- w145
      "Vds array" <- w144
      "corrected PD current array" <- w139
      "Ids array 2" <- w137
      "Corrected PD current array 2" <- w136
      "Vds array 2" <- w135
      "Vgs array 2" <- w134
      "Igs array 2" <- w133
      "?" <- w132
      n195 = Multiply(x=w123, y=sgl 5.0) -> (x*y=w130:sgl)
      n196 = local read "Loop"() -> (w141:bool)
      n197 = case shown="True" w141 {
        tunnel: w122 -> [w149 w153]
        tunnel: [w148 w151] -> w131
        frame False {
          n198 = Increment(x=w149) -> (x+1=w148:sgl)
        }
        frame True {
          n199 = Multiply(x=w153, y=sgl 2.0) -> (x*y=w150:sgl)
          n200 = Increment(x=w150) -> (x+1=w151:sgl)
        }
      }
      "Vds points" <- w131
      n201 = Initialize Array(0.0 ("element"), 0 ("dimension size")) -> (w126:dbl[])
      n202 = Build Array(w126) -> (w127:T2)
      n203 = Resize Matrix(1:w130, 2:w131, 4:w127) -> (0:→"data matrix":T2)
    }
    frame #4 {
      w346 = 0 items=["Set", "Get"] ("Operation (0: Set)")
      w348 = 1 items=["Current", "Voltage"] ("Source Mode (1: Voltage)")
      w345 = 1 items=["Channel 1", "Channel 2"] ("Channel (0: Channel 1)")
      w349 = 1 items=["Pulse", "DC"] ("Source Shape (1: DC)")
      w354 = 0 items=["Set", "Get"] ("Operation (0: Set)")
      w356 = 1 items=["Current", "Voltage"] ("Source Mode (1: Voltage)")
      w353 = 0 items=["Channel 1", "Channel 2"] ("Channel (0: Channel 1)")
      w357 = 1 items=["Pulse", "DC"] ("Source Shape (1: DC)")
      n204 = local read "Agilent address out"() -> (w337:refnum<visa-resource-name>)
      n205 = local read "error out agilent"() -> (w336:errorcluster)
      n206 = local read "light emission ON/OFF"() -> (w361:bool)
      n207 = case shown="True" w361 {
        frame False {
        }
        frame True {
          # "Turn 6487  off"
          n208 = local read "keithley address out"() -> (w363:refnum<k15>)
          n209 = local read "error out keithley"() -> (w362:errorcluster)
          n210 = call <instrlib>:"KE6485 Close.vi"("error in (no error)"=w362, "instrument handle"=w363) -> ("error out"=w364:errorcluster)  [unwired: 9 out]
          n211 = local write "error out keithley"(w364) -> ()
        }
      }
      n212 = call <instrlib>:"Configure Source.vi"("VISA resource name"=w337, "Channel (0: Channel 1)"=w353, "error in (no error)"=w336, "Source Shape (1: DC)"=w357, "Source Mode (1: Voltage)"=w356, "Output Level (0)"=0.0) -> ("VISA resource name out"=w359:refnum<visa-resource-name>, "error out"=w355:errorcluster)  [unwired: 12 in]
      n213 = call <instrlib>:"Enable Output.vi"("Enable Output (T: Enable)"=FALSE, "error in (no error)"=w355, "Operation (0: Set)"=w354, "Channel (0: Channel 1)"=w353, "VISA resource name"=w359) -> ("error out"=w343:errorcluster, "Output Enabled?"=w339:bool, "VISA resource name out"=w344:refnum<visa-resource-name>)  [unwired: 4 in]
      n214 = local write "channel 1 status"(w339) -> ()
      n215 = call <instrlib>:"Configure Source.vi"("VISA resource name"=w344, "Channel (0: Channel 1)"=w345, "error in (no error)"=w343, "Source Shape (1: DC)"=w349, "Source Mode (1: Voltage)"=w348, "Output Level (0)"=0.0) -> ("VISA resource name out"=w351:refnum<visa-resource-name>, "error out"=w347:errorcluster)  [unwired: 12 in]
      n216 = call <instrlib>:"Enable Output.vi"("Enable Output (T: Enable)"=FALSE, "error in (no error)"=w347, "Operation (0: Set)"=w346, "Channel (0: Channel 1)"=w345, "VISA resource name"=w351) -> ("error out"=w342:errorcluster, "Output Enabled?"=w340:bool, "VISA resource name out"=w341:refnum<visa-resource-name>)  [unwired: 4 in]
      n217 = local write "channel 2 status"(w340) -> ()
      n218 = call <instrlib>:"Close.vi"("error in (no error)"=w342, "VISA resource name"=w341) -> ("error out"=w338:errorcluster)  [unwired: 9 in]
      n219 = local write "error out agilent"(w338) -> ()
    }
    frame #5 {
      n220 = case shown="True" "AutoSave" {
        frame False {
          n221 = local read "corrected PD current array"() -> (w371:dbl[])
          n222 = local read "Vgs array"() -> (w372:dbl[])
          n223 = local read "Vgs array"() -> (w369:dbl[])
          n224 = local read "Ids array"() -> (w368:dbl[])
          n225 = local read "Igs array"() -> (w370:dbl[])
          n226 = Two Button Dialog(message="Do you want to save the data?") -> (T button?=w367:bool)  [unwired: 2 out]
          n227 = case shown="True" w367 {
            tunnel: w369 -> [_ w378]
            tunnel: w368 -> [_ w377]
            tunnel: w370 -> [_ w375]
            tunnel: w371 -> [_ w374]
            tunnel: w372 -> [_ w376]
            frame False {
            }
            frame True {
              n228 = Build Array(w376, w377, w378, w375, w374) -> ()  [unwired: 1 out]
              n229 = local read "data matrix"() -> (w373:dbl[][])
              n230 = call-poly <vilib>:"Write To Spreadsheet File.vi"("transpose? (no:F)"=TRUE, "format (%.3f)"="%.3e", "append to file? (new file:F)"=FALSE, "2D data"=w373) -> ()  [unwired: 4 in, 1 out]
            }
          }
        }
        frame True {
          w390 = "" ("delimiter (\\t)")
          n231 = call <vilib>:"Dflt Data Dir.vi"() -> ()  [unwired: 1 out]
          n232 = case shown="False" "WithTimeStamp" {
            tunnel: "File Name" -> [w393 w403]
            tunnel: [w392 w401] -> w387
            frame False {
              n233 = Format Into String(format string="%s.txt" ("Format string"), w393) -> (resulting string=w392:string)  [unwired: 2 in, 1 out]
            }
            frame True {
              n234 = Get Date/Time In Seconds() -> (seconds since 1Jan1904=w398:timestamp)
              n235 = Get Date/Time In Seconds() -> (seconds since 1Jan1904=w397:timestamp)
              n236 = Format Date/Time String(time format string (%c)="%Y%m%d" ("Timestamp string format i%cj"), seconds (now)=w398) -> (date/time string=w399:string)  [unwired: 1 out]
              n237 = Format Date/Time String(time format string (%c)="%H%M%S", seconds (now)=w397) -> (date/time string=w396:string)  [unwired: 1 out]
              n238 = Format Into String(format string="%s_%s_%s.txt" ("Format string"), w403, w399, w396) -> (resulting string=w401:string)  [unwired: 2 in, 1 out]
            }
          }
          n239 = Build Path(base path="File path", name or relative path=w387) -> (appended path=w386:path)
          n240 = local read "data matrix"() -> (w383:dbl[][])
          n241 = local read "header"() -> (w382:string[])
          n242 = call-poly <vilib>:"Write To Spreadsheet File.vi"("delimiter (\\t)"=w390, "1D data"=w382, "file path (dialog if empty)"=w386) -> ("new file path (Not A Path if cancelled)"=w385:path)  [unwired: 4 in, 1 out]
          n243 = call-poly <vilib>:"Write To Spreadsheet File.vi"("delimiter (\\t)"=w390, "append to file? (new file:F)"=TRUE, "2D data"=w383, "file path (dialog if empty)"=w385) -> ()  [unwired: 3 in, 2 out]
        }
      }
    }
  }
